vi "TCL Global.vi"() -> ()   [LabVIEW 2019]
panel:
  out "primary key":string
  out "current event file":path
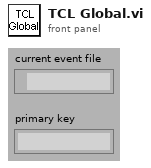
[diagram p1: front panel]
diagram:
